vi "Create Virtual Folder.vi"(8 "error in":errorcluster, 11 "project in":refnum<vi>) -> (0 "error out":errorcluster, 3 "virtual folder ref[]":refnum<vi>)   [LabVIEW 2021, in "Converter.lvlib"]
uses:
  Converter.lvlib
  Converter Reusables/Converter Reusables.lvlib
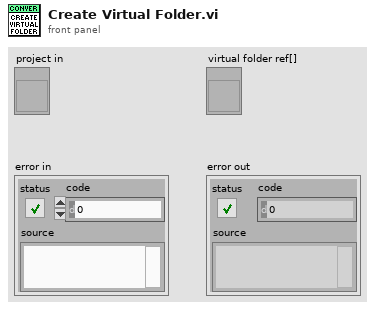
[diagram p1: front panel]
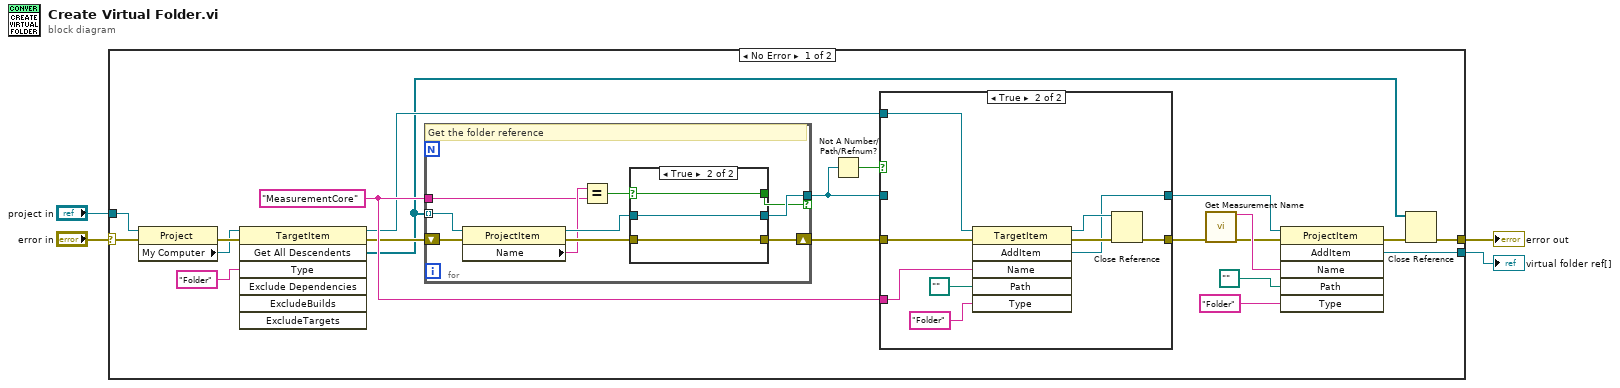
[diagram p0: block diagram]
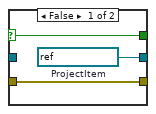
[diagram p2: hidden frame]
diagram:
  n1 = case shown="No Error" "error in" {
    selector: "error in" -> [w25 w53]
    tunnel: "project in" -> [w23 _]
    tunnel: [w20 _] -> w2
    tunnel: [w19 w53] -> w1
    frame No Error {
      w14 = "MeasurementCore" ("Name")
      n2 = property class="Project"(reference=w23, error in=w25) -> (error out=w24:errorcluster, "My Computer"=w12:refnum<vi>)  [unwired: 1 out]
      n3 = invoke class="TargetItem" method="Get All Descendents"(reference=w12, error in=w24, "Type"="Folder") -> (reference out=w10:refnum<vi>, error out=w11:errorcluster, "All Descendents"=w9:refnum<vi>[])  [unwired: 4 in, 4 out]
      n4 = for {
        tunnel: w9 -> [w35] mode=indexing
        shift-right: [w26] -> w15
        shift-left: w11 -> [w32]
        tunnel: w14 -> [w30]
        tunnel: [w28] -> w16 if=w27
        # "Get the folder reference"
        n5 = property class="ProjectItem"(reference=w35, error in=w32) -> (reference out=w33:refnum<vi>, error out=w34:errorcluster, "Name"=w31:string)
        n6 = Equal?(x=w31, y=w30) -> (x = y?=w29:bool)
        n7 = case shown="True" w29 {
          selector: w29 -> [w37 w40]
          tunnel: w34 -> [w38 w39]
          tunnel: w33 -> [_ w41]
          tunnel: [w36 w41] -> w28
          tunnel: [w37 w40] -> w27
          tunnel: [w38 w39] -> w26
          frame False {
            w36 = refnum<vi> refnum  # ProjectItem
          }
          frame True {
          }
        }
      }
      n8 = Not A Number/Path/Refnum?(number/path/refnum=w16) -> (NaN/Path/Refnum?=w18:bool)
      n9 = case shown="True" w18 {
        tunnel: [w43 w48] -> w17
        tunnel: w16 -> [w43 _]
        tunnel: w15 -> [w42 w47]
        tunnel: w14 -> [_ w46]
        tunnel: [w42 w45] -> w8
        tunnel: w10 -> [_ w44]
        frame False {
        }
        frame True {
          n10 = invoke class="TargetItem" method="AddItem"(reference=w44, error in=w47, "Name"=w46, "Path"=path "", "Type"="Folder") -> (reference out=w51:refnum<vi>, error out=w52:errorcluster, "AddItem"=w48:refnum<vi>)  [unwired: 1 in, 3 out]
          n11 = Close Reference(reference=w51, error in (no error)=w52) -> (error out=w45:errorcluster)
        }
      }
      n12 = call "Get Measurement Name.vi"("error in"=w8) -> ("name out"=w22:string, "error out"=w7:errorcluster)  [unwired: 13 in]
      n13 = invoke class="ProjectItem" method="AddItem"(reference=w17, error in=w7, "Name"=w22, "Path"=path "", "Type"="Folder") -> (error out=w21:errorcluster, "AddItem"=w20:refnum<vi>)  [unwired: 1 in, 4 out]
      n14 = Close Reference(reference=w9, error in (no error)=w21) -> (error out=w19:errorcluster)
    }
    frame Error {
    }
  }
  "error out" <- w1
  "virtual folder ref[]" <- w2
